vi "EncodeMessageFormat.vi"(0 "# of terminals":u8, 2 "CRef Types":T2[](array[typedef]), 3 "Terminal Bounds[]":T1[](array[typedef])) -> (5 "Messages":u8[](array[numeric]))   [LabVIEW 2012]
uses:
  CRef/Core/Master Types.ctl
  <vilib>/Utility/miscctls.llb/LVRectTypeDef.ctl
  CRef/CRef.lvlib
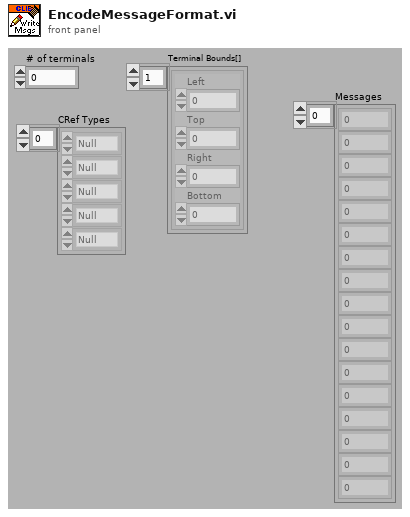
[diagram p1: front panel]
types:
  T1 = typedef "LVRectTypeDef.ctl" = cluster{"Left":i16, "Top":i16, "Right":i16, "Bottom":i16}
  T2 = typedef "CRef.lvlib/Master Types.ctl" = enum8{"Null", "Boolean", "U8", "I8", "U16", "I16", "U32", "I32", "U64", "I64", "Single", "Double", "Extended", "CSG", "CDB", "CXT", "Boolean(Def)", "U8(Def)", "I8(Def)", "U16(Def)", "I16(Def)", "U32(Def)", "I32(Def)", "Reserved Def", "Reserved Def1", "Single(Def)", "Double(Def)", "Reserved Def2", "Reserved Def3", "Reserved Def4", "Reserved Def5", "Unsigned(Def)", "Signed(Def)", "Real(Def)", "Reserved Def6", "Numeric(Def)", "String"}
  T3 = cluster{"Left":u8, "Top":u8, "Right":u8, "Bottom":u8}
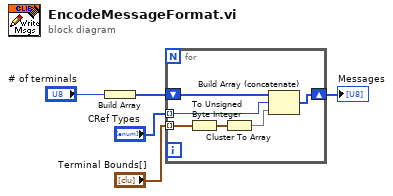
[diagram p0: block diagram]
diagram:
  n1 = Build Array("# of terminals") -> (w2:u8[])
  n2 = for {
    tunnel: "CRef Types" -> [w9] mode=indexing
    shift-right: [w8] -> w3
    shift-left: w2 -> [w7]
    tunnel: "Terminal Bounds[]" -> [w6] mode=indexing
    n3 = To Unsigned Byte Integer(number=w6) -> (unsigned 8bit integer=w11:T3)
    n4 = Cluster To Array(cluster=w11) -> (array=w10:u8[])
    n5 = Build Array (concatenate)(w7, w9, w10) -> (w8:u8[])
  }
  "Messages" <- w3
